vi "open data base.vi"() -> ()   [LabVIEW 2015]
uses:
  <vilib>/xnet/xnet.llb/XNET String To IO Name (Database Alias).vi
  <resource>/objmgr/xnet.rc
panel:
  out "Array 4":u32[](array[numeric]) format="%.0x"
  out "frames":string[](array[string])
  out "array of filepath":path[](array[path])
  out "array of alias":string[](array[string])
  out "Array 3":string[](array[string])
  out "Array 2":u32[](array[numeric])
  out "Array":string[](array[string])
  in  "Path":path
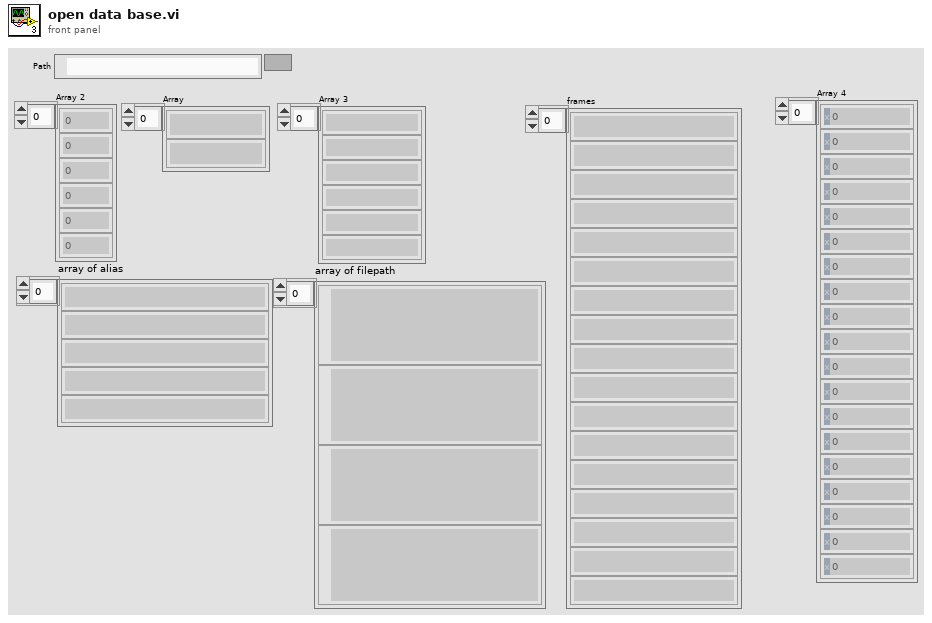
[diagram p1: front panel]
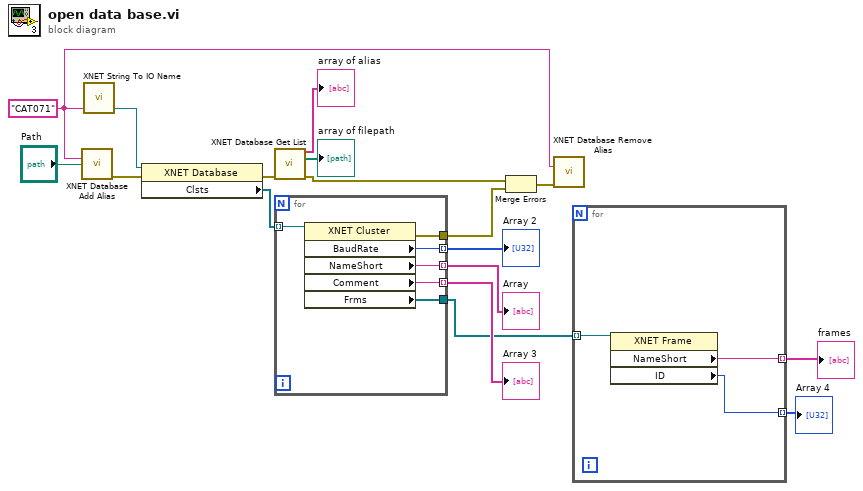
[diagram p0: block diagram]
diagram:
  w4 = "CAT071" ("string")
  n1 = call <vilib>:"XNET Database Add Alias.vi"("alias"=w4, "filepath"="Path") -> ("error out"=w10:errorcluster)  [unwired: 13 in]
  n2 = call-poly <vilib>:"XNET String To IO Name.vi"("string"=w4) -> ("XNET Database"=w8:refnum<k21>)  [unwired: 4 out]
  n3 = property class="XNET Database"(reference=w8, error in=w10) -> (error out=w13:errorcluster, "Clsts"=w17:refnum<k21>[])  [unwired: 1 out]
  n4 = call <vilib>:"XNET Database Get List.vi"("error in (no error)"=w13) -> ("array of alias"=→"array of alias":string[], "array of filepath"=→"array of filepath":path[], "error out"=w5:errorcluster)  [unwired: 12 in]
  n5 = for {
    tunnel: w17 -> [w23] mode=indexing
    tunnel: [w22] -> w16 mode=indexing
    tunnel: [w21] -> w15 mode=indexing
    tunnel: [w20] -> w14 mode=indexing
    tunnel: [w19] -> w7
    tunnel: [w18] -> w3
    n6 = property class="XNET Cluster"(reference=w23) -> (error out=w19:errorcluster, "BaudRate"=w21:u32, "NameShort"=w22:string, "Comment"=w20:string, "Frms"=w18:refnum<k21>[])  [unwired: 1 in, 1 out]
  }
  "Array" <- w16
  "Array 2" <- w15
  "Array 3" <- w14
  n7 = Merge Errors(w5, w7) -> (w6:errorcluster)
  n8 = call <vilib>:"XNET Database Remove Alias.vi"("alias"=w4, "error in (no error)"=w6) -> ()  [unwired: 13 in, 1 out]
  n9 = for {
    tunnel: w3 -> [w26] mode=indexing
    tunnel: [w25] -> w2 mode=indexing
    tunnel: [w24] -> w1 mode=indexing
    n10 = property class="XNET Frame"(reference=w26) -> ("NameShort"=w25:string, "ID"=w24:u32)  [unwired: 1 in, 2 out]
  }
  "frames" <- w2
  "Array 4" <- w1
